vi "View AO param.vi"(7 "ActivateAIView":bool, 9 "AO in":T1, 11 "AOTable":dbl[](array[numeric]) format="%#.0f") -> (2 "Reread out":bool, 3 "This VI":refnum<vi>)   [LabVIEW 2019, in "Inputs.lvlib"]
uses:
  Inputs.lvlib
  Ctl/AO.ctl
  Ctl/Parameter State.ctl
  Database/Progress.vi
  Database/PostgreSQL.lvlib
  Logik/Logik.lvlib
panel:
  out "AO progress":i32(slide) scale=0.0..100.0
  in  "Reread":bool
  in  "n_elem":i32(c297)
  out "units":string[](array[string])
  out "AO_9":dbl format="%#.1f"
  out "AO_10":dbl format="%#.1f"
  out "AO_5":dbl format="%#.1f"
  out "AO_6":dbl format="%#.1f"
  out "AO_7":dbl format="%#.1f"
  out "AO_8":dbl format="%#.1f"
  out "AO_3":dbl format="%#.1f"
  out "AO_4":dbl format="%#.1f"
  out "AO_2":dbl format="%#.1f"
  out "AO_1":dbl format="%#.1f"
  out "n param":i32
  out "Names":string[](array[string])
  out "parameters":string[](array[string])
  out "Parameters table":dbl[][](array[numeric])=[[1.0, 0.0, 1000.0, 2.0, 0.0, 0.0, 2.0, 20.0, 100.0, nan, 250.0, 250.0, 2.0, 1.0, 10.0, 0.0, 65535.0, 0.0, 250.0, 1.0, 4.0], [1.0, 0.0, 1000.0, 2.0, 0.0, 0.0, 2.0, 20.0, 150.0, nan, 250.0, 250.0, 2.0, 1.0, 11.0, 0.0, 65535.0, 0.0, 250.0, 0.0, 4.0], [1.0, 0.0, 1000.0, 2.0, 0.0, 0.0, 2.0, 3.0, 7.0, 8.0, 10.0, 10.0, 2.0, 0.1, 1.0, 0.0, 65535.0, 0.0, 10.0, 0.0, 2.0], [1.0, 0.0, 1000.0, 2.0, 0.0, 0.0, 1.5, 2.5, 6.0, 7.0, 10.0, 10.0, 2.0, 0.1, 2.0, 0.0, 65535.0, 0.0, 10.0, 0.0, 3.0], [1.0, 0.0, 1000.0, 2.0, 0.0, 0.0, 2.0, 2.5, 6.0, 7.0, 10.0, 10.0, 2.0, 0.1, 3.0, 0.0, 65535.0, 0.0, 10.0, 1.0, 2.0], [1.0, 0.0, 1000.0, 2.0, 0.0, 0.0, 1.5, 2.0, 4.0, 5.0, 10.0, 10.0, 2.0, 0.1, 4.0, 0.0, 65535.0, 0.0, 10.0, 1.0, 3.0], [1.0, 0.0, 1000.0, 2.0, 0.0, 0.0, 3.0, 4.0, 8.0, 9.0, 10.0, 10.0, 2.0, 0.1, 5.0, 0.0, 65535.0, 0.0, 100.0, 1.0, 7.0], [1.0, 0.0, 1000.0, 2.0, 0.0, 0.0, 4.0, 8.0, nan, nan, 100.0, 100.0, 2.0, 1.0, 6.0, 0.0, 65535.0, 0.0, 100.0, 0.0, 0.0], [1.0, 0.0, 1000.0, 2.0, 0.0, 0.0, nan, nan, nan, nan, 100.0, 100.0, 2.0, 1.0, 7.0, 0.0, 65535.0, 0.0, 100.0, 0.0, 1.0], [1.0, 0.0, 1000.0, 2.0, 0.0, 0.0, nan, nan, nan, nan, 100.0, 100.0, 2.0, 1.0, 8.0, 0.0, 65535.0, 0.0, 100.0, 1.0, 0.0], [1.0, 0.0, 1000.0, 2.0, 0.0, 0.0, 10.0, 15.0, 45.0, 50.0, 100.0, 100.0, 2.0, 1.0, 9.0, 0.0, 65535.0, 0.0, 100.0, 1.0, 1.0]]
  # "instrument_range_max"
  # "instrument_range_min"
  # "output_pv_min"
  # "output_pv_max"
  # "output_register_min"
  # "output_register_max"
  # "control_channel_num"
  # "module_num"
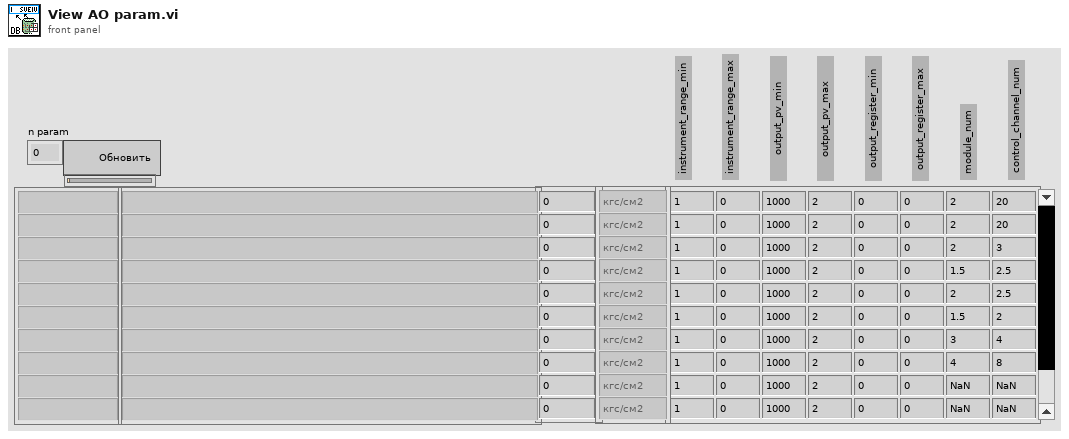
[diagram p1: front panel]
types:
  T1 = typedef "Inputs.lvlib/AO.ctl" = cluster{"AO_defs":cluster{"AO_def":dbl[], "AOint_def":u16[][], "AOState_def":T2[], "AOALRState_def":errorcluster[]}, "modified":refnum<data-value>, "AOP":refnum<data-value>, "AONames":refnum<data-value>}
  T2 = typedef "Inputs.lvlib/Parameter State.ctl" = cluster{"code":i32, "visible":bool, "color":u32, "source":string}
  T3 = enum32{"Invalid", "Standard", "Closed", "Hidden", "Minimized", "Maximized"}
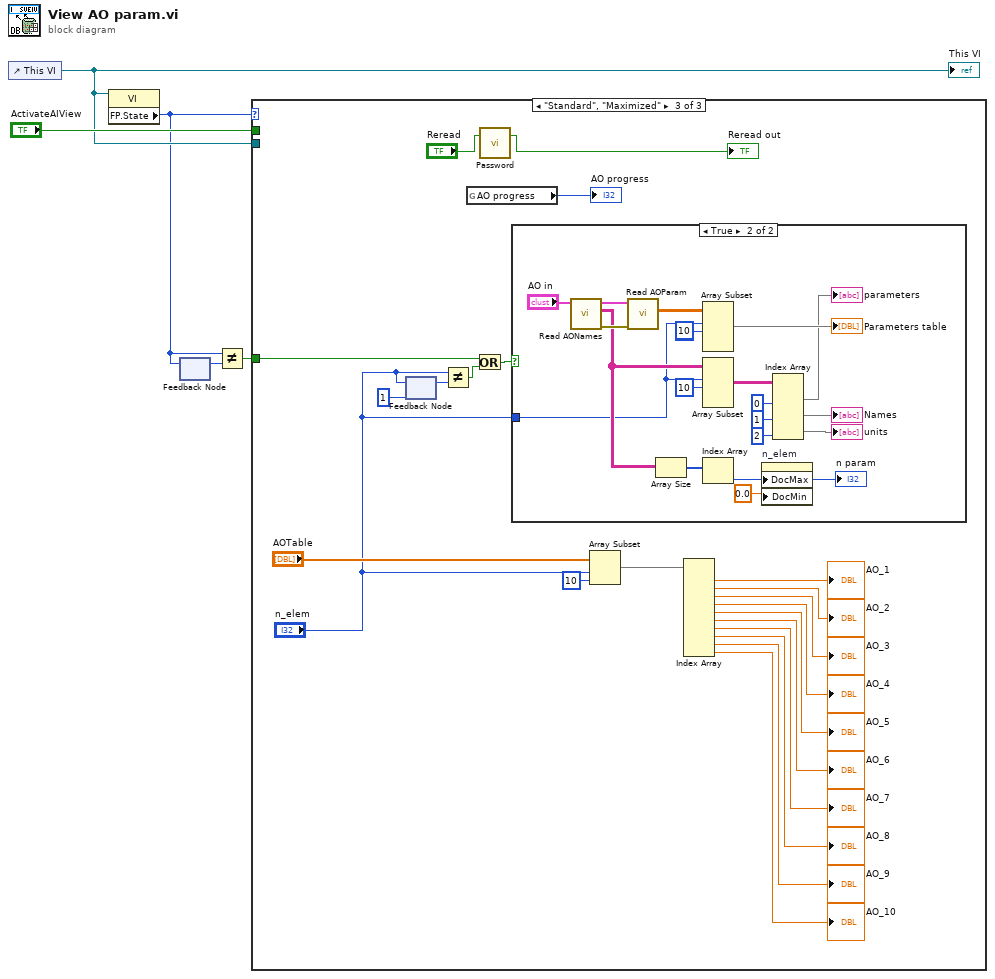
[diagram p0: block diagram]
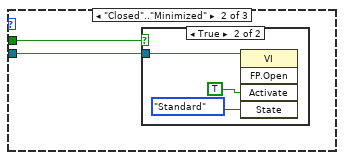
[diagram p3: hidden frame]
diagram:
  n1 = control-ref of="This VI"() -> (w4:refnum<vi>)
  "This VI" <- w4
  n2 = property class="VI"(reference=w4) -> ("FP.State"=w1:T3)  [unwired: 1 in, 2 out]
  n3 = feedback #1() -> (w3:T3)  [unwired: 1 in]
  n4 = feedback-in #1(w1) -> ()
  n5 = Not Equal?(x=w1, y=w3) -> (x != y?=w2:bool)
  n6 = case shown="\"Standard\", \"Maximized\"" w1 {
    tunnel: "ActivateAIView" -> [_ w7 _]
    tunnel: w4 -> [_ w6 _]
    tunnel: w2 -> [_ _ w11]
    frame "Invalid", Default {
    }
    frame "Closed".."Minimized" {
      n7 = case shown="True" w7 {
        tunnel: w6 -> [_ w8]
        frame False {
        }
        frame True {
          n8 = invoke class="VI" method="FP.Open"(reference=w8, "Activate"=TRUE ("Activate?"), "State"=T3."Standard") -> ()  [unwired: 2 in, 5 out]
        }
      }
    }
    frame "Standard", "Maximized" {
      n9 = feedback #2(1 ("n_elem")) -> (w16:i32)
      n10 = feedback-in #2("n_elem") -> ()
      n11 = Not Equal?(x="n_elem", y=w16) -> (x != y?=w15:bool)
      n12 = global read "Progress.vi" "AO progress"() -> (→"AO progress":i32)
      n13 = Or(x=w11, y=w15) -> (x .or. y?=w13:bool)
      n14 = call "Password.vi"("ActivatePASSWView"="Reread") -> ("enable"=→"Reread out":bool)  [unwired: 1 in, 1 out]
      n15 = case shown="True" w13 {
        tunnel: "n_elem" -> [_ w33]
        frame False {
        }
        frame True {
          (unwired) 10 ("length")
          n16 = call "Read AONames.vi"("AO in"="AO in") -> ("error out"=w46:errorcluster, "AONames"=w37:string[][], "AO out"=w45:T1)  [unwired: 8 in]
          n17 = call "Read AOParam.vi"("error in (no error)"=w46, "AO in"=w45) -> ("AOParam"=w44:dbl[][])  [unwired: 7 in, 2 out]
          n18 = Array Size(array=w37) -> (size(s)=w35:i32[])
          n19 = Array Subset(array=w44, index (row)=w33, length (row)=10 ("length")) -> (→"Parameters table":dbl[][])  [unwired: 2 in]
          n20 = Array Subset(array=w37, index (row)=w33, length (row)=10 ("length")) -> (w42:string[][])  [unwired: 2 in]
          n21 = Index Array(array=w35) -> (element=w34:i32)  [unwired: 1 in]
          "n param" <- w34
          n22 = property on="n_elem" class="Scroll (strict)"("DocMax"=w34, "DocMin"=0.0 ("Data Entry Limits:Minimum")) -> ()  [unwired: 2 in, 2 out]
          n23 = Index Array(array=w42, index (col) #1=0 ("disabled index (col)"), index (col) #2=1 ("disabled index (col)"), index (col) #3=2 ("disabled index (col)")) -> (element #1=→"parameters":string[], element #2=→"Names":string[], element #3=→"units":string[])  [unwired: 3 in]
        }
      }
      n24 = Array Subset(array="AOTable", index="n_elem", length=10) -> (w21:dbl[])
      n25 = Index Array(array=w21) -> (element #1=→"AO_1":dbl, element #2=→"AO_2":dbl, element #3=→"AO_3":dbl, element #4=→"AO_4":dbl, element #5=→"AO_5":dbl, element #6=→"AO_6":dbl, element #7=→"AO_7":dbl, element #8=→"AO_8":dbl, element #9=→"AO_9":dbl, element #10=→"AO_10":dbl)  [unwired: 10 in]
    }
  }
